vi "Array_Index_To_Colour.vi"(1 "Formation=False":bool[][](array[boolean])=[[TRUE, TRUE, TRUE, TRUE, TRUE, TRUE, TRUE, TRUE, TRUE, TRUE], [TRUE, TRUE, TRUE, TRUE, TRUE, TRUE, TRUE, TRUE, TRUE, TRUE], [FALSE, FALSE, TRUE, TRUE, TRUE, TRUE, TRUE, TRUE, TRUE, TRUE], [TRUE, TRUE, TRUE, TRUE, FALSE, FALSE, FALSE, FALSE, FALSE, FALSE], [TRUE, TRUE, TRUE, TRUE, TRUE, TRUE, TRUE, TRUE, TRUE, TRUE], [TRUE, TRUE, TRUE, TRUE, TRUE, TRUE, TRUE, TRUE, TRUE, TRUE], [TRUE, TRUE, TRUE, TRUE, TRUE, TRUE, TRUE, TRUE, TRUE, TRUE], [TRUE, TRUE, TRUE, TRUE, TRUE, TRUE, FALSE, FALSE, FALSE, FALSE], [FALSE, FALSE, FALSE, FALSE, FALSE, FALSE, FALSE, FALSE, TRUE, TRUE], [TRUE, TRUE, FALSE, FALSE, FALSE, FALSE, TRUE, TRUE, TRUE, TRUE]], 2 "Horizontal dim size":i32, 3 "Vertical dim size":i32, 4 "Cap Module Number":i32[][](array[numeric])=[[43, 44, 45, 46, 47, 48, 0, 0, 0, 0], [33, 34, 35, 36, 37, 38, 39, 40, 41, 42], [71, 72, 25, 26, 27, 28, 29, 30, 31, 32], [61, 62, 63, 64, 65, 66, 67, 68, 69, 70], [51, 52, 53, 54, 55, 56, 57, 58, 59, 60], [49, 50, 92, 96, 17, 21, 20, 24, 89, 93], [1, 2, 3, 4, 5, 6, 7, 8, 73, 74], [75, 76, 77, 78, 79, 80, 81, 82, 83, 84], [9, 10, 11, 12, 13, 14, 15, 16, 18, 19], [22, 23, 85, 86, 87, 88, 90, 91, 94, 95]], 5 "Threshold":i32, 6 "Slider Index":i32, 7 "Chart History":dbl[][](array[numeric])) -> (0 "Cap Voltages":cluster{"Color Box":u32, "Numeric":i32}[][](array[cluster])=[[{"Color Box"=16775416, "Numeric"=0}, {"Color Box"=16775673, "Numeric"=0}, {"Color Box"=16775930, "Numeric"=0}, {"Color Box"=16775930, "Numeric"=0}, {"Color Box"=16773103, "Numeric"=0}, {"Color Box"=16774131, "Numeric"=0}, {"Color Box"=16774388, "Numeric"=0}, {"Color Box"=16774388, "Numeric"=0}, {"Color Box"=16775159, "Numeric"=0}, {"Color Box"=16775673, "Numeric"=0}], [{"Color Box"=16773874, "Numeric"=0}, {"Color Box"=16774131, "Numeric"=0}, {"Color Box"=16775159, "Numeric"=0}, {"Color Box"=16774645, "Numeric"=0}, {"Color Box"=16777215, "Numeric"=0}, {"Color Box"=16777215, "Numeric"=0}, {"Color Box"=16777215, "Numeric"=0}, {"Color Box"=16777215, "Numeric"=0}, {"Color Box"=16777215, "Numeric"=0}, {"Color Box"=16777215, "Numeric"=0}], [{"Color Box"=16449530, "Numeric"=71}, {"Color Box"=16580604, "Numeric"=72}, {"Color Box"=16777215, "Numeric"=0}, {"Color Box"=16777215, "Numeric"=0}, {"Color Box"=16777215, "Numeric"=0}, {"Color Box"=16777215, "Numeric"=0}, {"Color Box"=16777215, "Numeric"=0}, {"Color Box"=16777215, "Numeric"=0}, {"Color Box"=16777215, "Numeric"=0}, {"Color Box"=16777215, "Numeric"=0}], [{"Color Box"=16776187, "Numeric"=61}, {"Color Box"=16775673, "Numeric"=62}, {"Color Box"=16776187, "Numeric"=63}, {"Color Box"=16515067, "Numeric"=64}, {"Color Box"=16515067, "Numeric"=65}, {"Color Box"=16515067, "Numeric"=66}, {"Color Box"=16318456, "Numeric"=67}, {"Color Box"=16318456, "Numeric"=68}, {"Color Box"=16449530, "Numeric"=69}, {"Color Box"=16318456, "Numeric"=70}], [{"Color Box"=16775159, "Numeric"=51}, {"Color Box"=16775159, "Numeric"=52}, {"Color Box"=16775930, "Numeric"=53}, {"Color Box"=16775930, "Numeric"=54}, {"Color Box"=16776444, "Numeric"=55}, {"Color Box"=16775159, "Numeric"=56}, {"Color Box"=16776187, "Numeric"=57}, {"Color Box"=16775930, "Numeric"=58}, {"Color Box"=16776187, "Numeric"=59}, {"Color Box"=16775930, "Numeric"=60}], [{"Color Box"=16775159, "Numeric"=49}, {"Color Box"=16774388, "Numeric"=50}, {"Color Box"=16776701, "Numeric"=92}, {"Color Box"=16776187, "Numeric"=96}, {"Color Box"=16770276, "Numeric"=17}, {"Color Box"=16773103, "Numeric"=21}, {"Color Box"=16774645, "Numeric"=20}, {"Color Box"=16775673, "Numeric"=24}, {"Color Box"=16776444, "Numeric"=89}, {"Color Box"=16775416, "Numeric"=93}], [{"Color Box"=16775416, "Numeric"=1}, {"Color Box"=16775159, "Numeric"=2}, {"Color Box"=16775159, "Numeric"=3}, {"Color Box"=16773103, "Numeric"=4}, {"Color Box"=16774902, "Numeric"=5}, {"Color Box"=16775930, "Numeric"=6}, {"Color Box"=16775673, "Numeric"=7}, {"Color Box"=16772332, "Numeric"=8}, {"Color Box"=16776187, "Numeric"=73}, {"Color Box"=16776701, "Numeric"=74}], [{"Color Box"=16776187, "Numeric"=75}, {"Color Box"=16776444, "Numeric"=76}, {"Color Box"=16776444, "Numeric"=77}, {"Color Box"=16776187, "Numeric"=78}, {"Color Box"=16776444, "Numeric"=79}, {"Color Box"=16776444, "Numeric"=80}, {"Color Box"=16383993, "Numeric"=81}, {"Color Box"=16515067, "Numeric"=82}, {"Color Box"=16449530, "Numeric"=83}, {"Color Box"=16515067, "Numeric"=84}], [{"Color Box"=15794160, "Numeric"=9}, {"Color Box"=15400938, "Numeric"=10}, {"Color Box"=14680031, "Numeric"=11}, {"Color Box"=15859697, "Numeric"=12}, {"Color Box"=16252919, "Numeric"=13}, {"Color Box"=15794160, "Numeric"=14}, {"Color Box"=11141033, "Numeric"=15}, {"Color Box"=15990771, "Numeric"=16}, {"Color Box"=16776444, "Numeric"=18}, {"Color Box"=16734553, "Numeric"=19}], [{"Color Box"=16773360, "Numeric"=22}, {"Color Box"=16775930, "Numeric"=23}, {"Color Box"=15466475, "Numeric"=85}, {"Color Box"=16449530, "Numeric"=86}, {"Color Box"=16580604, "Numeric"=87}, {"Color Box"=16515067, "Numeric"=88}, {"Color Box"=16776444, "Numeric"=90}, {"Color Box"=16775930, "Numeric"=91}, {"Color Box"=16776701, "Numeric"=94}, {"Color Box"=16776444, "Numeric"=95}]])   [LabVIEW 2016]
doc: "Converts integer array elements to the intensity of a colour box. The output array contains a cluster of the colour box and an extra identifying number. The output colour can be either green or red, based on an internal boolean array."
panel:
  out "32bit integer":i32[][](array[numeric])
  out "Testing Array 2":dbl[][](array[numeric])
  out "Testing Array":dbl[][](array[numeric])
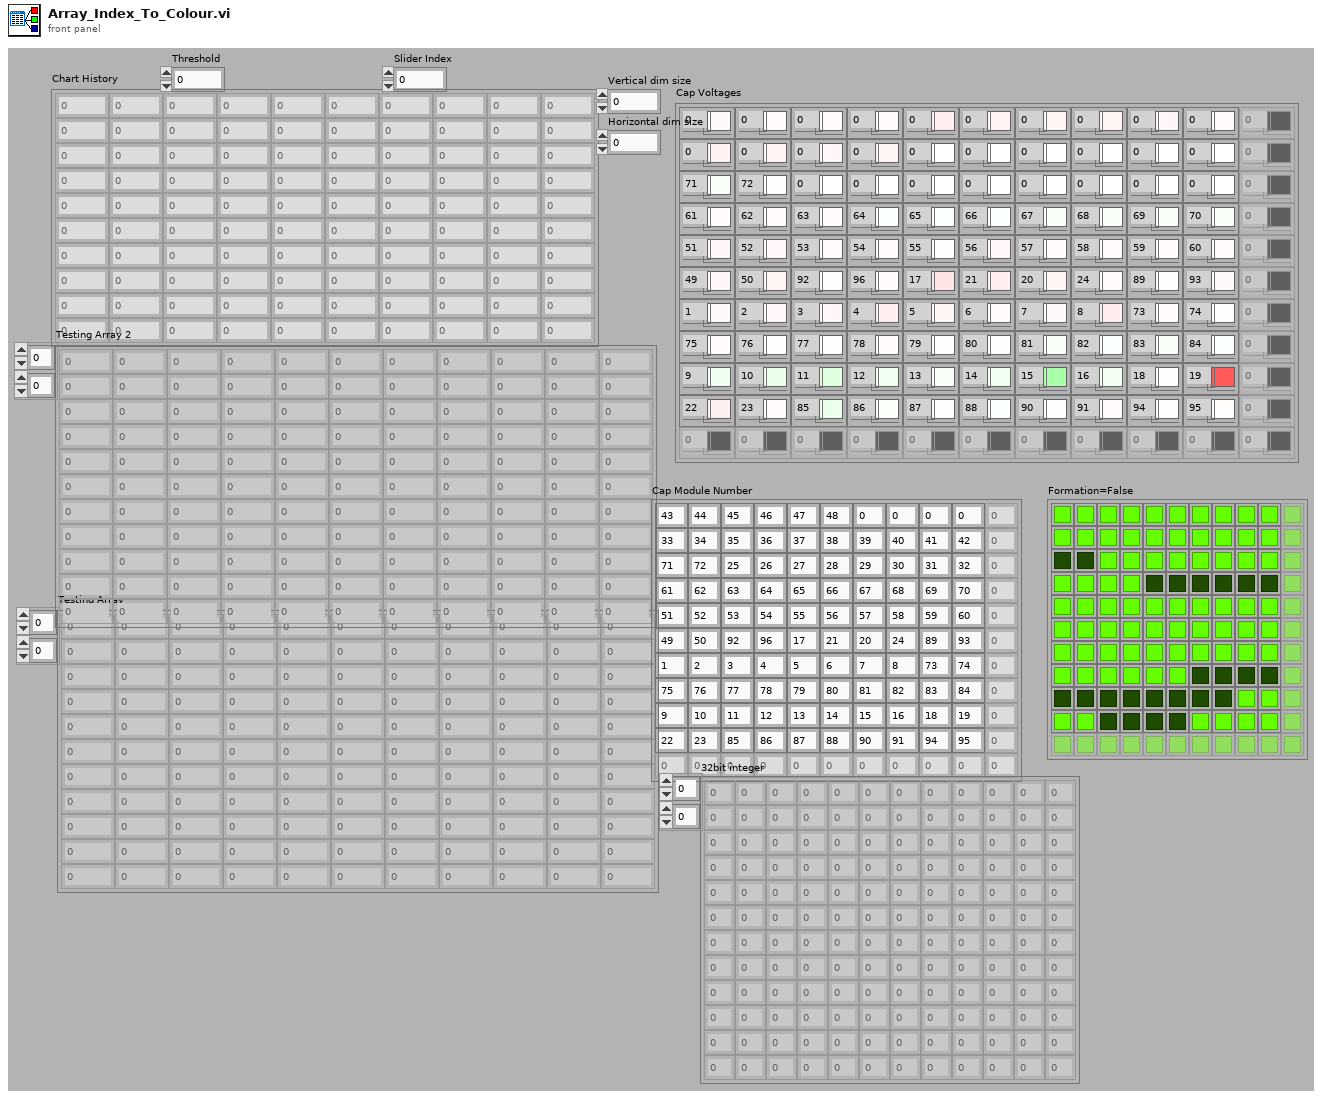
[diagram p1: front panel]
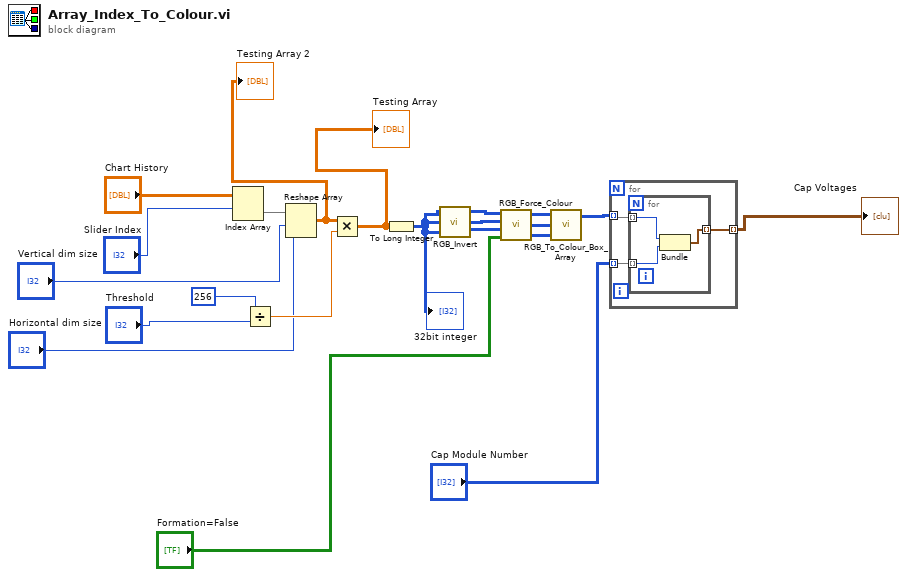
[diagram p0: block diagram]
diagram:
  n1 = Index Array(array="Chart History", index (row)="Slider Index") -> (element=w21:dbl[])  [unwired: 1 in]
  n2 = Divide(x=256, y="Threshold") -> (x/y=w19:dbl)
  n3 = Reshape Array(w21, "Vertical dim size", "Horizontal dim size") -> (w4:dbl[][])
  "Testing Array 2" <- w4
  n4 = Multiply(x=w4, y=w19) -> (x*y=w5:dbl[][])
  "Testing Array" <- w5
  n5 = To Long Integer(number=w5) -> (32bit integer=w14:i32[][])
  "32bit integer" <- w14
  n6 = call "RGB_Invert.vi"("Blue"=w14, "Green"=w14, "Red"=w14) -> ("Invert Blue"=w11:i32[][], "Invert Green"=w12:i32[][], "Invet Red"=w13:i32[][])
  n7 = call "RGB_Force_Colour.vi"("Red or Green Force"="Formation=False", "Blue"=w11, "Green"=w12, "Red"=w13) -> ("Forced Blue"=w7:i32[][], "Forced Green"=w8:i32[][], "Forced Red"=w9:i32[][])
  n8 = call "RGB_To_Colour_Box_Array.vi"("Blue"=w7, "Green"=w8, "Red"=w9) -> ("Colour Box"=w6:u32[][])
  n9 = for {
    tunnel: "Cap Module Number" -> [w23] mode=indexing
    tunnel: w6 -> [w24] mode=indexing
    tunnel: [w22] -> w18 mode=indexing
    n10 = for {
      tunnel: w24 -> [w27] mode=indexing
      tunnel: w23 -> [w26] mode=indexing
      tunnel: [w25] -> w22 mode=indexing
      n11 = Bundle("Color Box"=w27, w26) -> (w25:cluster{"Color Box":u32, i32})  [unwired: 1 in]
    }
  }
  "Cap Voltages" <- w18
